vi "SendToDb.vi"(0 "reference in":refnum<class "DI.lvclass">, 11 "error in (no error)":errorcluster) -> (4 "reference out":refnum<class "DI.lvclass">, 15 "error out":errorcluster)   [LabVIEW 2019, in "DI.lvclass"]
uses:
  DI.lvclass
  D:/GIT H4000/H4000/src/Proccess_class/Proccess.lvclass
  Proccess_class/Proccess.lvclass/Proccess.ctl
  DI.lvclass/DI.ctl
  Logger_class/EventData.ctl
  TypeDef/AlarmType.ctl
  Logger_class/Logger.lvclass
  Proccess_class/Proccess.lvclass
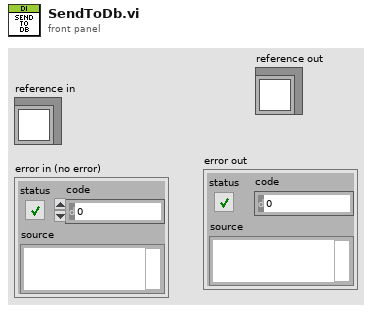
[diagram p1: front panel]
types:
  T1 = typedef "EventData.ctl" = cluster{"obj_tag":string, "event_tag":string, "Description":string, "ALARM TYPE":T2, "Value DBL":dbl, "Value INT":i32, "Value STR":string, "Time Stamp":timestamp}
  T2 = typedef "AlarmType.ctl" = enum16{"Normal", "Warning", "Alarm"}
  T3 = typedef "Proccess.lvclass/TAGs.ctl" = cluster{"TAG":string, "PTAG":string, "DESC":string}
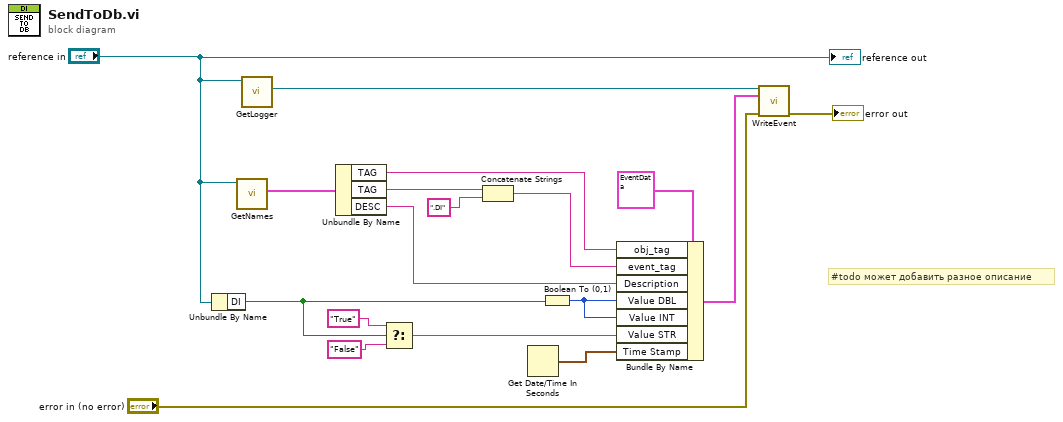
[diagram p0: block diagram]
diagram:
  # "#todo может добавить разное описание"
  n1 = Unbundle By Name("reference in") -> ("DI"=w1:bool)
  n2 = call "GetNames.vi"("Proccess in"="reference in") -> ("Tags"=w10:T3)  [unwired: 10 in]
  n3 = call "GetLogger.vi"("Proccess in"="reference in") -> ("Logger"=w12:refnum<class "Logger.lvclass">)  [unwired: 10 in]
  n4 = Unbundle By Name(w10) -> ("TAG"=w9:string, "TAG"=w8:string, "DESC"=w7:string)
  n5 = Select(t="True" ("Value STR"), s=w1, f="False") -> (s? t:f=w3:string)
  n6 = Concatenate Strings(w8, ".DI" ("string")) -> (w14:string)
  n7 = Get Date/Time In Seconds() -> (seconds since 1Jan1904=w2:timestamp)
  n8 = Boolean To (0,1)(Boolean=w1) -> (0, 1=w6:i16)
  n9 = Bundle By Name(cluster=T1 {"obj_tag"="", "event_tag"="", "Description"="", "ALARM TYPE"=enum."Normal", "Value DBL"=0.0, "Value INT"=0, "Value STR"="", "Time Stamp"=timestamp(0 s since 1904-01-01)} ("Event"), "obj_tag"=w9, "event_tag"=w14, "Description"=w7, "Value DBL"=w6, "Value INT"=w6, "Value STR"=w3, "Time Stamp"=w2) -> (w16:T1)
  n10 = call "WriteEvent.vi"("reference in"=w12, "Event"=w16, "error in (no error)"="error in (no error)") -> ("error out"=→"error out":errorcluster)  [unwired: 11 in, 1 out]
  "reference out" <- "reference in"
